vi "set gear settings.vi"(8 "error in (no error)":errorcluster, 10 "gear_settings":T1, 11 "id":i32) -> (0 "error out":errorcluster, 3 "function return":i32)   [LabVIEW 2012, in "libximc.lvlib"]
doc: "result_t XIMC_API set_gear_settings (device_t id, const gear_settings_t* gear_settings);"
uses:
  libximc.lvlib
  libximc.dll
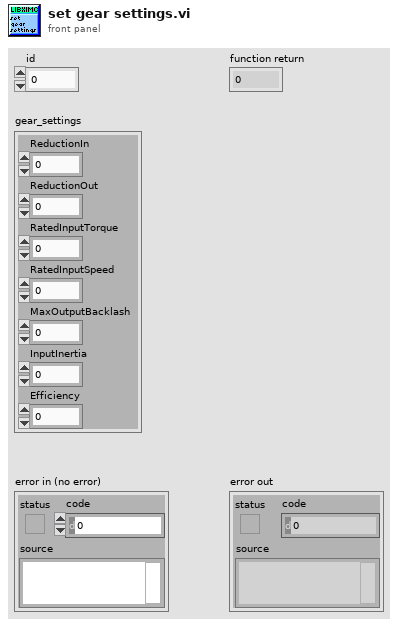
[diagram p1: front panel]
types:
  T1 = cluster{"ReductionIn":sgl, "ReductionOut":sgl, "RatedInputTorque":sgl, "RatedInputSpeed":sgl, "MaxOutputBacklash":sgl, "InputInertia":sgl, "Efficiency":sgl}
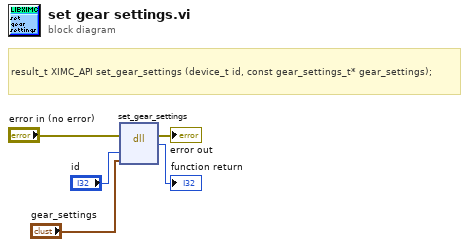
[diagram p0: block diagram]
diagram:
  # "result_t XIMC_API set_gear_settings (device_t id, const gear_settings_t* gear_settings);"
  n1 = dll-call lib="C:/Users/Stepan/Downloads/labview_2.9.11_testgen_thread/libximc.*" fn="set_gear_settings"(error in="error in (no error)", "id"="id", "gear_settings"="gear_settings") -> (error out=→"error out":errorcluster, →"function return":i32)  [unwired: 4 in, 1 out]
